vi "Start_Timer.vi"(8 "error in (no error)":errorcluster, 11 "Timer_Event in":refnum<class "Timer_Event.lvclass">) -> (0 "error out":errorcluster, 3 "Timer_Event out":refnum<class "Timer_Event.lvclass">)   [LabVIEW 2020, in "Timer_Event.lvlib" / "Timer_Event.lvclass"]
uses:
  Timer_Event.lvclass
  Timer_Event.lvclass/Timer_Event.ctl
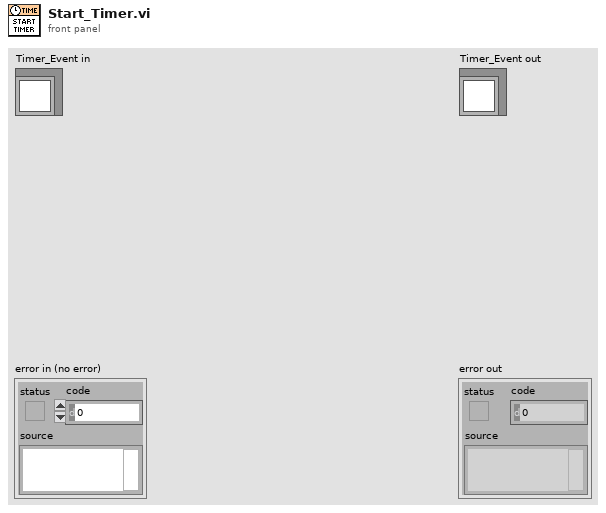
[diagram p1: front panel]
types:
  T1 = cluster{"Start Time":i32, "Elapsed Time":i32, "Running?":bool}
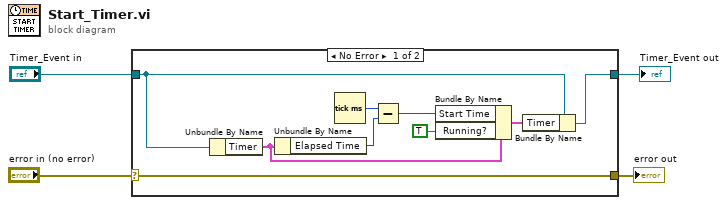
[diagram p0: block diagram]
diagram:
  n1 = case shown="No Error" "error in (no error)" {
    selector: "error in (no error)" -> [w13 w15]
    tunnel: [w13 w15] -> w3
    tunnel: [w5 w14] -> w1
    tunnel: "Timer_Event in" -> [w6 w14]
    frame No Error {
      n2 = Unbundle By Name(w6) -> ("Timer"=w9:T1)
      n3 = Unbundle By Name(w9) -> ("Elapsed Time"=w8:i32)
      n4 = Tick Count (ms)() -> (millisecond timer value=w10:u32)
      n5 = Subtract(x=w10, y=w8) -> (x-y=w11:u32)
      n6 = Bundle By Name(cluster=w9, "Start Time"=w11, "Running?"=TRUE ("Running")) -> (w7:T1)
      n7 = Bundle By Name(cluster=w6, "Timer"=w7) -> (w5:refnum<class "Timer_Event.lvclass">)
    }
    frame Error {
    }
  }
  "error out" <- w3
  "Timer_Event out" <- w1
